vi "Memory.Pointer.Read.Safe.1D.SGL.vi"(8 "error in (no error)":errorcluster, 9 "count":u64 format="%d elements", 10 "buffer in":sgl[](array[numeric]), 11 "pointer in":refnum<class "Memory.Pointer.lvclass">) -> (0 "error out":errorcluster, 1 "count out":u64 format="%d elements", 2 "buffer out":sgl[](array[numeric]), 3 "pointer out":refnum<class "Memory.Pointer.lvclass">)   [LabVIEW 2016, in "Memory Manager.lvlib" / "Memory.Pointer.lvclass"]
doc: "Reads <b>count</b> elements from the address specified by <b>pointer</b> into the provided <b>buffer</b>.\n\n<b>Note:</b> This VI is <b>unsafe</b>.\n\nUnsafe means that it does not evaluate the size parameter of <b>pointer</b> to ensure that is inbounds of allocated memory before peforming a memory read/write. Reading/writing more data to a pointer than it has allocated can corrupt or crash LabVIEW. Only use this VI in scenarios where the <b>pointer</b> has been validated to be allocated to a correct size before calling this VI."
uses:
  Memory.Pointer.lvclass
  Memory.Pointer.lvclass/Memory.Pointer.ctl
  Accessors/Get Address.vi
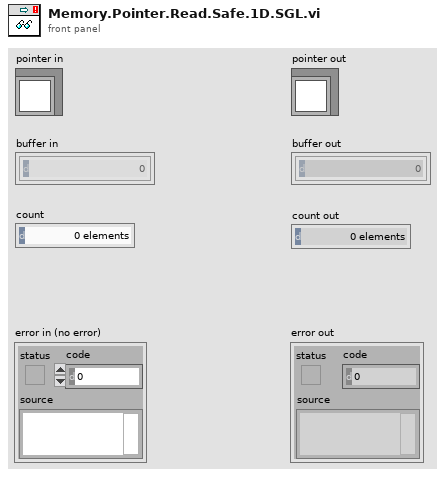
[diagram p1: front panel]
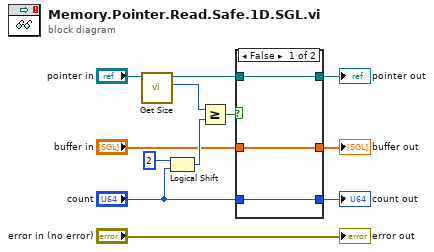
[diagram p0: block diagram]
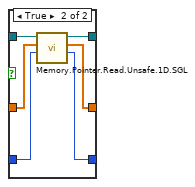
[diagram p2: hidden frame]
diagram:
  n1 = call "Get Size.vi"("Pointer in"="pointer in") -> ("size"=w9:u64, "Pointer out"=w7:refnum<class "Memory.Pointer.lvclass">)  [unwired: 8 in, 1 out]
  n2 = Logical Shift(y=i16 2, x="count") -> (x << y=w10:u64)
  n3 = Greater Or Equal?(x=w9, y=w10) -> (x >= y?=w8:bool)
  n4 = case shown="False" w8 {
    tunnel: w7 -> [w15 w21]
    tunnel: [w15 w20] -> w6
    tunnel: "buffer in" -> [w14 w19]
    tunnel: "count" -> [w13 w18]
    tunnel: [w14 w17] -> w2
    tunnel: [w13 w16] -> w1
    frame False {
    }
    frame True {
      n5 = call "Memory.Pointer.Read.Unsafe.1D.SGL.vi"("count"=w18, "buffer in"=w19, "pointer in"=w21) -> ("count out"=w16:u64, "buffer out"=w17:sgl[], "pointer out"=w20:refnum<class "Memory.Pointer.lvclass">)  [unwired: 5 in, 1 out]
    }
  }
  "pointer out" <- w6
  "buffer out" <- w2
  "count out" <- w1
  "error out" <- "error in (no error)"
